vi "Get Debug Mode.vi"(8 "error in (no error)":errorcluster, 11 "SMO":refnum<class "SMO.lvclass">) -> (0 "error out":errorcluster, 2 "Behavior":T1, 3 "SMO out":refnum<class "SMO.lvclass">)   [LabVIEW 2019, in "Debug.lvlib"]
uses:
  Debug.lvlib
  <vilib>/JKI/JKI SMO/SMO/SMO.lvclass
  Attribute.Debug/DebugBehavior.ctl
  Attribute.Debug/Attribute.Debug.lvclass/Attribute.Debug.ctl
  SMO.Mediator/SMO.Mediator.lvclass
  Attribute.Debug/Attribute.Debug.lvclass
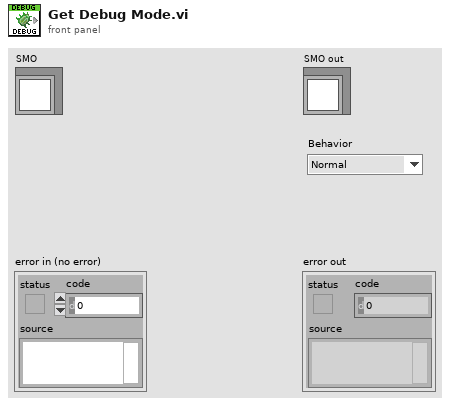
[diagram p1: front panel]
types:
  T1 = typedef "Debug.lvlib/Attribute.Debug.lvclass/DebugBehavior.ctl" = enum16{"Normal", "Debug"}
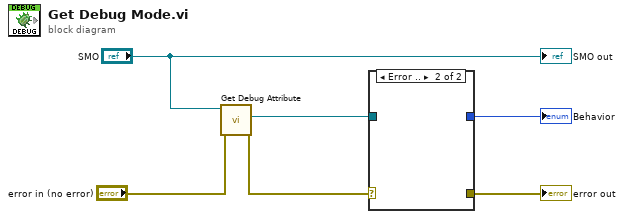
[diagram p0: block diagram]
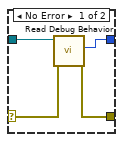
[diagram p2: hidden frame]
diagram:
  n1 = call "Get Debug Attribute.vi"("error in (no error)"="error in (no error)", "SMO"="SMO") -> ("error out"=w3:errorcluster, "Attribute.Debug"=w4:refnum<class "Attribute.Debug.lvclass">)  [unwired: 7 in, 1 out]
  n2 = case shown="Error .." w3 {
    selector: w3 -> [w9 _]
    tunnel: w4 -> [w10 _]
    tunnel: [w8 _] -> w2
    tunnel: [w7 _] -> w1
    frame No Error {
      n3 = call "Read Debug Behavior.vi"("error in (no error)"=w9, "Attribute.Debug in"=w10) -> ("error out"=w8:errorcluster, "Behavior"=w7:T1)  [unwired: 7 in, 1 out]
    }
    frame Error {
    }
  }
  "error out" <- w2
  "Behavior" <- w1
  "SMO out" <- "SMO"
